vi "crop-images.vi"() -> ()   [LabVIEW 2014]
uses:
  <vilib>/vision/NI_Vision_Development_Module.lvlib
panel:
  in  "Save Image?":bool
  in  "Start Path":path
  in  "Cancel":bool
  out "Cropped Image":T1(plugin-control)
  in  "Crop":bool
  out "Original Image":T1(plugin-control)
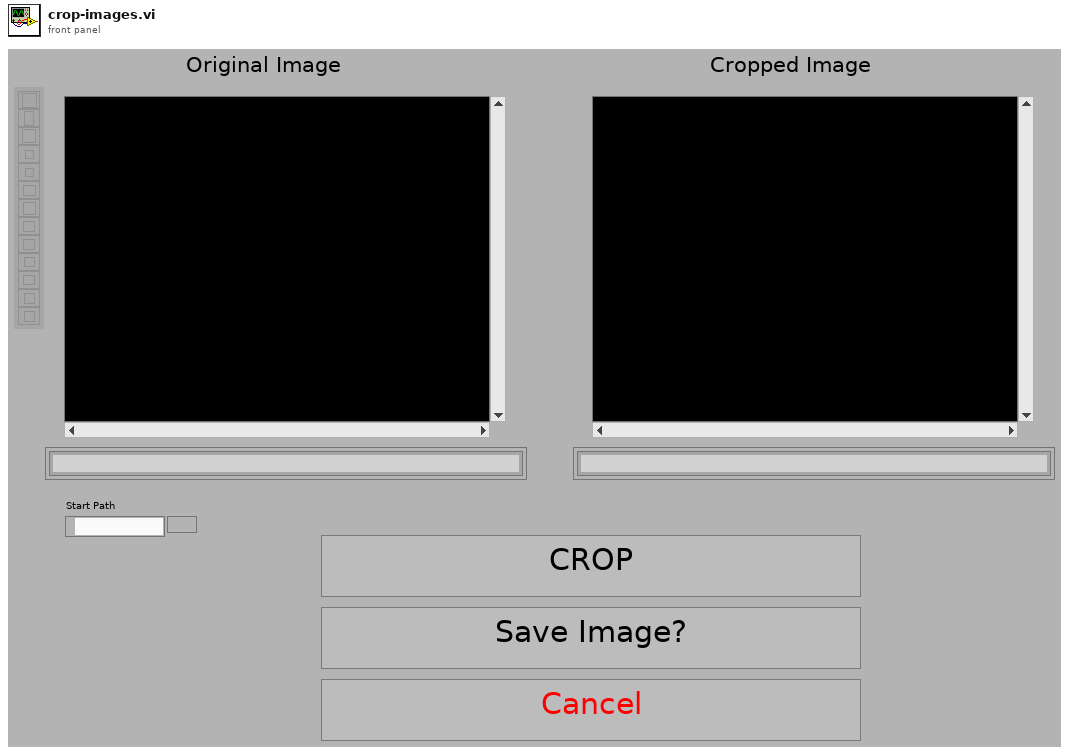
[diagram p1: front panel]
types:
  T1 = typedef "IMAQ Image.ctl" = refnum<image>
  T2 = typedef "Image Type" = u32
  T3 = cluster{"Global Rectangle":i32[], "Contours":cluster{"Contour Type":u32, "ROI Type":u32, "Points":i32[]}[]}
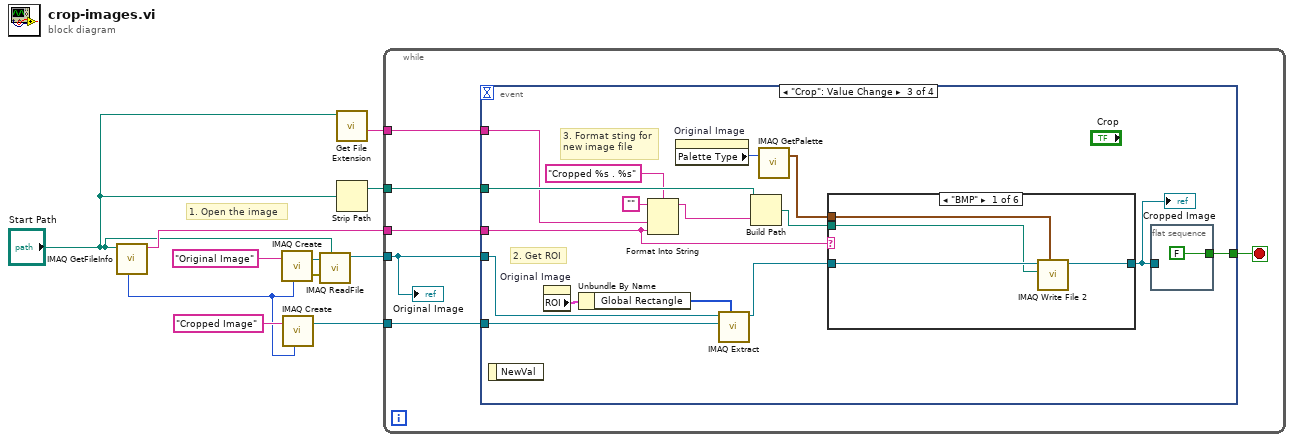
[diagram p0: block diagram]
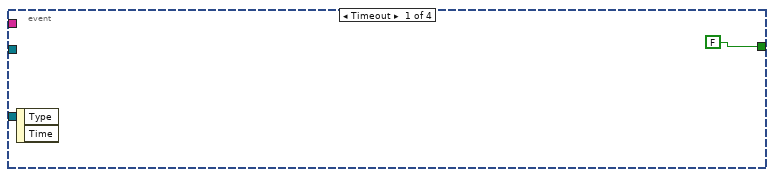
[diagram p2: hidden frame]
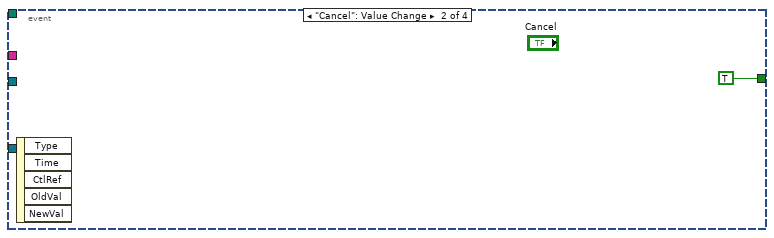
[diagram p3: hidden frame]
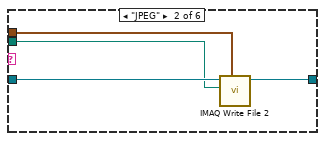
[diagram p4: hidden frame]
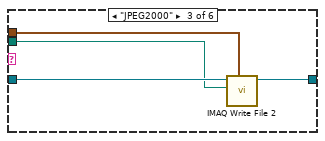
[diagram p5: hidden frame]
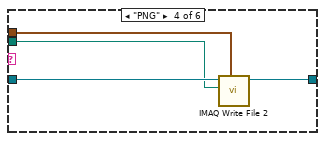
[diagram p6: hidden frame]
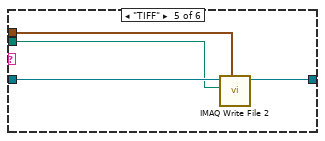
[diagram p7: hidden frame]
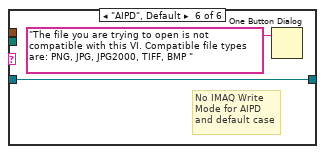
[diagram p8: hidden frame]
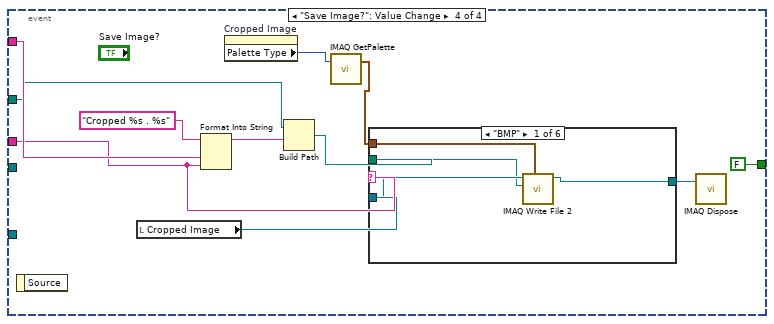
[diagram p9: hidden frame]
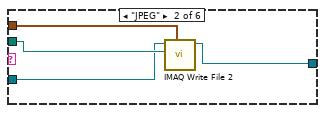
[diagram p10: hidden frame]
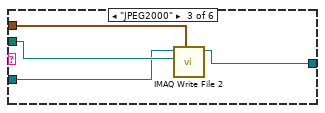
[diagram p11: hidden frame]
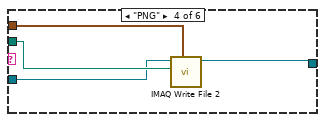
[diagram p12: hidden frame]
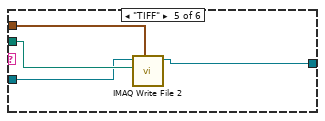
[diagram p13: hidden frame]
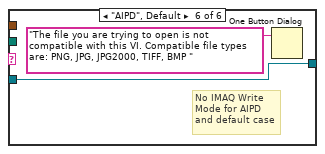
[diagram p14: hidden frame]
diagram:
  # "1. Open the image"
  n1 = call "IMAQ GetFileInfo"("File Path"="Start Path") -> ("File Type"=w4:string, "Image Type"=w5:T2)  [unwired: 4 in, 5 out]
  n2 = call "IMAQ Create"("Image Name"="Original Image", "Image Type"=w5) -> ("New Image"=w11:T1, "error out"=w2:errorcluster)  [unwired: 3 in]
  n3 = call "IMAQ Create"("Image Name"="Cropped Image", "Image Type"=w5) -> ("New Image"=w7:T1)  [unwired: 3 in, 1 out]
  n4 = call "IMAQ ReadFile"("File Path"="Start Path", "error in (no error)"=w2, "Image"=w11) -> ("Image Out"=w8:T1)  [unwired: 4 in, 4 out]
  n5 = call <vilib>:"Get File Extension.vi"("file"="Start Path") -> ("filename without extension"=w3:string)  [unwired: 7 in, 3 out]
  n6 = Strip Path(path="Start Path") -> (stripped path=w6:path)  [unwired: 1 out]
  n7 = while {
    tunnel: w8 -> [w17]
    tunnel: w7 -> [w16]
    tunnel: w6 -> [w14]
    tunnel: w4 -> [w13]
    tunnel: w3 -> [w12]
    stop <- w15 stop-if-true
    n8 = event shown="[2] \"Crop\": Value Change" {
      selector: _ -> [_ _ _ _]
      dyn-events: _ -> [_ _ _ _]
      timeout: _ -> [_ _ _ _]
      tunnel: w17 -> [_ _ w34 _]
      tunnel: w16 -> [_ _ w33 _]
      tunnel: [FALSE TRUE w35 FALSE] -> w15
      tunnel: w14 -> [_ _ w29 w66]
      tunnel: w13 -> [_ _ w23 w65]
      tunnel: w12 -> [_ _ w20 w68]
      event Timeout {
        n9 = event-data() -> ()  [unwired: 1 in, 2 out]
      }
      event "Cancel": Value Change {
        n10 = event-data() -> ()  [unwired: 1 in, 5 out]
      }
      event "Crop": Value Change {
        # "3. Format sting for new image file"
        # "2. Get ROI"
        n11 = event-data() -> ()  [unwired: 1 in, 1 out]
        n12 = property on="Original Image" class="ImageControl"() -> ("ROI"=w32:T3)  [unwired: 2 in, 2 out]
        n13 = Unbundle By Name(w32) -> ("Global Rectangle"=w31:i32[])
        n14 = Format Into String(format string="Cropped %s . %s", initial string="", w20, w23) -> (resulting string=w22:string)  [unwired: 1 in, 1 out]
        n15 = property on="Original Image" class="ImageControl"() -> ("Palette Type"=w26:u32)  [unwired: 2 in, 2 out]
        n16 = call "IMAQ Extract"("Optional Rectangle"=w31, "Image Dst"=w33, "Image Src"=w34) -> ("Image Dst Out"=w30:T1)  [unwired: 7 in, 1 out]
        n17 = Build Path(base path=w29, name or relative path=w22) -> (appended path=w28:path)
        n18 = call "IMAQ GetPalette"("Palette Number (gray)"=w26) -> ("Color Palette"=w27:cluster{"Red":u8, "Green":u8, "Blue":u8}[])  [unwired: 4 in, 1 out]
        n19 = case shown="\"BMP\"" w23 {
          tunnel: [w39 w43 w47 w51 w55 w57] -> w21
          tunnel: w30 -> [w38 w42 w46 w50 w54 w57]
          tunnel: w28 -> [w37 w41 w45 w49 w53 _]
          tunnel: w27 -> [w36 w40 w44 w48 w52 _]
          frame "BMP" {
            n20 = call-poly "IMAQ Write File 2"("Color Palette"=w36, "File Path"=w37, "Image"=w38) -> ("Image Out (duplicate)"=w39:T1)  [unwired: 7 in, 1 out]
          }
          frame "JPEG" {
            n21 = call-poly "IMAQ Write File 2"("Color Palette"=w40, "File Path"=w41, "Image"=w42) -> ("Image Out (duplicate)"=w43:T1)  [unwired: 7 in, 1 out]
          }
          frame "JPEG2000" {
            n22 = call-poly "IMAQ Write File 2"("Color Palette"=w44, "File Path"=w45, "Image"=w46) -> ("Image Out (duplicate)"=w47:T1)  [unwired: 7 in, 1 out]
          }
          frame "PNG" {
            n23 = call-poly "IMAQ Write File 2"("Color Palette"=w48, "File Path"=w49, "Image"=w50) -> ("Image Out (duplicate)"=w51:T1)  [unwired: 7 in, 1 out]
          }
          frame "TIFF" {
            n24 = call-poly "IMAQ Write File 2"("Color Palette"=w52, "File Path"=w53, "Image"=w54) -> ("Image Out (duplicate)"=w55:T1)  [unwired: 7 in, 1 out]
          }
          frame "AIPD", Default {
            # "No IMAQ Write Mode for AIPD and default case"
            n25 = One Button Dialog(message="The file you are trying to open is not compatible with this VI. Compatible file types are: PNG, JPG, JPG2000, TIFF, BMP ") -> ()  [unwired: 1 in, 1 out]
          }
        }
        "Cropped Image" <- w21
        n26 = flat-sequence {
          tunnel: [FALSE] -> w35
          tunnel: w21 -> [_]
          frame #0 {
          }
        }
      }
      event "Save Image?": Value Change {
        n27 = event-data() -> ()  [unwired: 1 in, 1 out]
        n28 = local read "Cropped Image"() -> (w64:T1)
        n29 = Format Into String(initial string="Cropped %s . %s" ("format string"), w68, w65) -> (resulting string=w67:string)  [unwired: 2 in, 1 out]
        n30 = property on="Cropped Image" class="ImageControl"() -> ("Palette Type"=w60:u32)  [unwired: 2 in, 2 out]
        n31 = Build Path(base path=w66, name or relative path=w67) -> (appended path=w63:path)
        n32 = call "IMAQ GetPalette"("Palette Number (gray)"=w60) -> ("Color Palette"=w59:cluster{"Red":u8, "Green":u8, "Blue":u8}[])  [unwired: 4 in, 1 out]
        n33 = case shown="\"BMP\"" w65 {
          tunnel: w64 -> [w73 w76 w80 w84 w88 w90]
          tunnel: w63 -> [w72 w77 w81 w85 w89 _]
          tunnel: [w71 w75 w79 w83 w87 w90] -> w61
          tunnel: w59 -> [w70 w74 w78 w82 w86 _]
          frame "BMP" {
            n34 = call-poly "IMAQ Write File 2"("Color Palette"=w70, "File Path"=w72, "Image"=w73) -> ("Image Out (duplicate)"=w71:T1)  [unwired: 7 in, 1 out]
          }
          frame "JPEG" {
            n35 = call-poly "IMAQ Write File 2"("Color Palette"=w74, "File Path"=w77, "Image"=w76) -> ("Image Out (duplicate)"=w75:T1)  [unwired: 7 in, 1 out]
          }
          frame "JPEG2000" {
            n36 = call-poly "IMAQ Write File 2"("Color Palette"=w78, "File Path"=w81, "Image"=w80) -> ("Image Out (duplicate)"=w79:T1)  [unwired: 7 in, 1 out]
          }
          frame "PNG" {
            n37 = call-poly "IMAQ Write File 2"("Color Palette"=w82, "File Path"=w85, "Image"=w84) -> ("Image Out (duplicate)"=w83:T1)  [unwired: 7 in, 1 out]
          }
          frame "TIFF" {
            n38 = call-poly "IMAQ Write File 2"("Color Palette"=w86, "File Path"=w89, "Image"=w88) -> ("Image Out (duplicate)"=w87:T1)  [unwired: 7 in, 1 out]
          }
          frame "AIPD", Default {
            # "No IMAQ Write Mode for AIPD and default case"
            n39 = One Button Dialog(message="The file you are trying to open is not compatible with this VI. Compatible file types are: PNG, JPG, JPG2000, TIFF, BMP ") -> ()  [unwired: 1 in, 1 out]
          }
        }
        n40 = call "IMAQ Dispose"("Image"=w61) -> ()  [unwired: 5 in, 1 out]
      }
    }
    "Original Image" <- w17
  }
